vi "Move.vi"(1 "Right":T3={"PowerRight"=80, "RotationRight(Degrees)"=360, "PortRight"=2} {"PortRight" items=["Port A"=0, "Port B"=1, "Port C"=2, "Ports A & B"=4, "Ports A & C"=5, "Ports B & C"=6, "All Ports"=3]}, 2 "Left":T2={"PowerLeft"=100, "RotationLeft(Degrees)"=360, "PortLeft"=1} {"PortLeft" items=["Port A"=0, "Port B"=1, "Port C"=2, "Ports A & B"=4, "Ports A & C"=5, "Ports B & C"=6, "All Ports"=3]}, 3 "BrickReference in":T4) -> (0 "BrickReference out":T4)   [LabVIEW 2015]
uses:
  <vilib>/NXT/Subs/LVHSConnector.ctl
  <vilib>/NXT/LegoClasses/BrickReference/BrickReference.lvclass
  <vilib>/NXT/Subs/MotorOutput.ctl
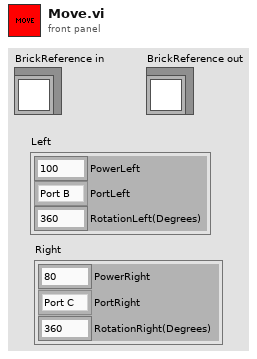
[diagram p1: front panel]
types:
  T1 = typedef "MotorOutput.ctl" = u8
  T2 = cluster{"PowerLeft":i32, "RotationLeft(Degrees)":i32, "PortLeft":T1}
  T3 = cluster{"PowerRight":i32, "RotationRight(Degrees)":i32, "PortRight":T1}
  T4 = typedef "LVHSConnector.ctl" = refnum<class "BrickReference.lvclass">
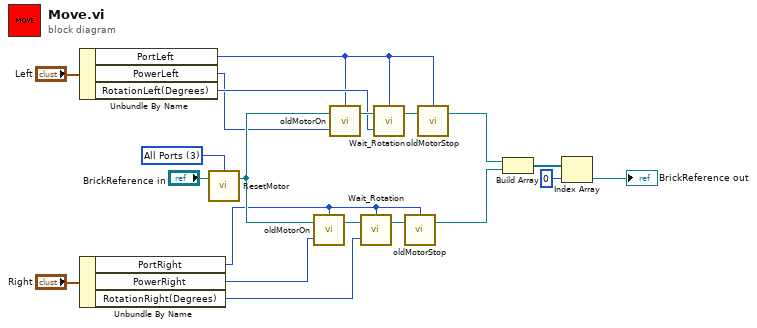
[diagram p0: block diagram]
diagram:
  w19 = T1 3 items=["Port A"=0, "Port B"=1, "Port C"=2, "Ports A & B"=4, "Ports A & C"=5, "Ports B & C"=6, "All Ports"=3] ("Port (All Ports)")
  n1 = Unbundle By Name("Left") -> ("PortLeft"=w4:T1, "PowerLeft"=w5:i32, "RotationLeft(Degrees)"=w6:i32)
  n2 = Unbundle By Name("Right") -> ("PortRight"=w3:T1, "PowerRight"=w2:i32, "RotationRight(Degrees)"=w1:i32)
  n3 = call <vilib>:"ResetMotor.vi"("NXT/EV3"="BrickReference in", "Port (All Ports)"=w19) -> ("NXT/EV3"=w14:T4)  [unwired: 2 in]
  n4 = call <vilib>:"oldMotorOn.vi"("Power (75)"=w2, "NXT/EV3"=w14, "Output Port (All Ports)"=w3) -> ("NXT/EV3"=w18:T4)  [unwired: 1 in]
  n5 = call <vilib>:"oldMotorOn.vi"("Power (75)"=w5, "NXT/EV3"=w14, "Output Port (All Ports)"=w4) -> ("NXT/EV3"=w16:T4)  [unwired: 1 in]
  n6 = call <vilib>:"Wait_Rotation.vi"("Position Change (180)"=w1, "NXT/EV3"=w18, "Port (Port A)"=w3) -> ("NXT/EV3"=w17:T4)  [unwired: 1 in]
  n7 = call <vilib>:"Wait_Rotation.vi"("Position Change (180)"=w6, "NXT/EV3"=w16, "Port (Port A)"=w4) -> ("NXT/EV3"=w15:T4)  [unwired: 1 in]
  n8 = call <vilib>:"oldMotorStop.vi"("NXT/EV3"=w17, "Output Port (All Ports)"=w3) -> ("NXT/EV3"=w12:T4)  [unwired: 2 in]
  n9 = call <vilib>:"oldMotorStop.vi"("NXT/EV3"=w15, "Output Port (All Ports)"=w4) -> ("NXT/EV3"=w13:T4)  [unwired: 2 in]
  n10 = Build Array(w13, w12) -> (w11:T4[])
  n11 = Index Array(array=w11, index=0) -> (element=→"BrickReference out":T4)
